vi "NegI64.vi"(4 "x":i64) -> (1 "-x":i64, 2 "Overflow?":bool)   [LabVIEW 2017, in "GPOverflow.lvlib"]
doc: "Negates <B>x</B> keeping track of numeric overflow.\n\n<B>Overflow?</B> will be True if positive or negative overflow occurred. The output will saturate in case of overflow.\n\nThis VI is inlined.\n\nSteen Schmidt\nGPower\n8/8 2013"
uses:
  GPOverflow.lvlib
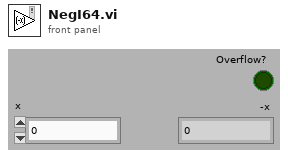
[diagram p1: front panel]
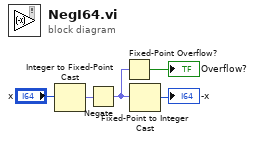
[diagram p0: block diagram]
diagram:
  n1 = Integer to Fixed-Point Cast(integer="x") -> (fixed-point=w1:fxp<+/-,64,64>)  [unwired: 1 in]
  n2 = Negate(x=w1) -> (-x=w4:fxp<+/-,64,64>)
  n3 = Fixed-Point Overflow?(1:w4) -> (0:→"Overflow?":bool)
  n4 = Fixed-Point to Integer Cast(1:w4) -> (0:→"-x":i64)
